vi "Get as LabVIEW Text.vi"(8 "error in (no error)":errorcluster, 10 "Name Array":string[](array[string]), 11 "JSON Running Mean In":refnum<class "JSON Running Mean.lvclass">) -> (0 "error out":errorcluster, 1 "Was in quotes":bool, 2 "LabVIEW Text":string, 3 "JSON Running Mean Out":refnum<class "JSON Running Mean.lvclass">)   [LabVIEW 2020, in "Library Commun.lvlib" / "JSON Running Mean.lvclass"]
uses:
  JSON Running Mean.lvclass
  JSON Value/JSON Value.lvclass
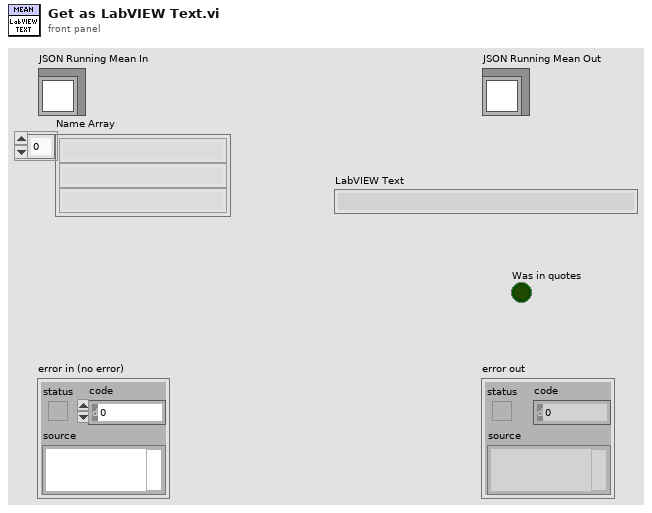
[diagram p1: front panel]
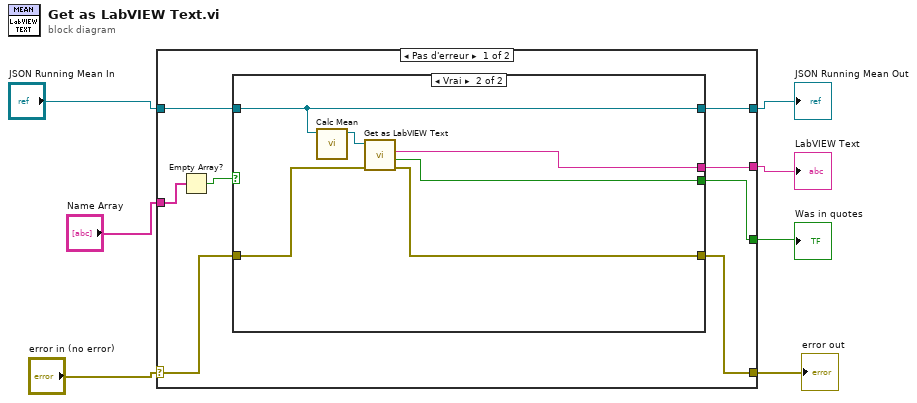
[diagram p0: block diagram]
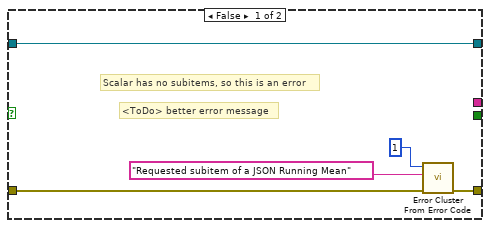
[diagram p2: hidden frame]
diagram:
  n1 = case shown="Pas d'erreur" "error in (no error)" {
    selector: "error in (no error)" -> [w10 w28]
    tunnel: [w9 w28] -> w3
    tunnel: [w11 w27] -> w6
    tunnel: "JSON Running Mean In" -> [w12 w27]
    tunnel: [w15 _] -> w1
    tunnel: "Name Array" -> [w14 _]
    tunnel: [w8 _] -> w2
    frame No Error {
      n2 = Empty Array?(array=w14) -> (empty?=w13:bool)
      n3 = case shown="Vrai" w13 {
        tunnel: w12 -> [w20 w26]
        tunnel: [_ w24] -> w15
        tunnel: [w20 w26] -> w11
        tunnel: w10 -> [w16 w21]
        tunnel: [w19 w22] -> w9
        tunnel: [_ w23] -> w8
        frame False {
          # "<ToDo> better error message"
          # "Scalar has no subitems, so this is an error"
          n4 = call <vilib>:"Error Cluster From Error Code.vi"("error in (no error)"=w16, "error message (\"\")"="Requested subitem of a JSON Running Mean" ("error message (\"\")"), "error code (0)"=1) -> ("error out"=w19:errorcluster)  [unwired: 6 in]
        }
        frame True {
          n5 = call-dynamic "Calc Mean.vi"("JSON Statistics in"=w26) -> ("JSON Value"=w25:refnum<class "JSON Value.lvclass">)  [unwired: 10 in]
          n6 = call-dynamic "Get as LabVIEW Text.vi"("error in (no error)"=w21, "JSON Value In"=w25) -> ("error out"=w22:errorcluster, "Was in quotes"=w23:bool, "LabVIEW Text"=w24:string)  [unwired: 6 in, 1 out]
        }
      }
    }
    frame Error {
    }
  }
  "error out" <- w3
  "JSON Running Mean Out" <- w6
  "LabVIEW Text" <- w1
  "Was in quotes" <- w2
